vi "Free.vi"(8 "error in (no error)":errorcluster, 11 "Object (subject) in":refnum<class "Object (subject).lvclass">) -> (0 "error out":errorcluster, 3 "Object (subject) out":refnum<class "Object (subject).lvclass">)   [LabVIEW 2014, in "Object (subject).lvclass"]
uses:
  Object (subject).lvclass
  Object (subject).lvclass/Object (subject).ctl
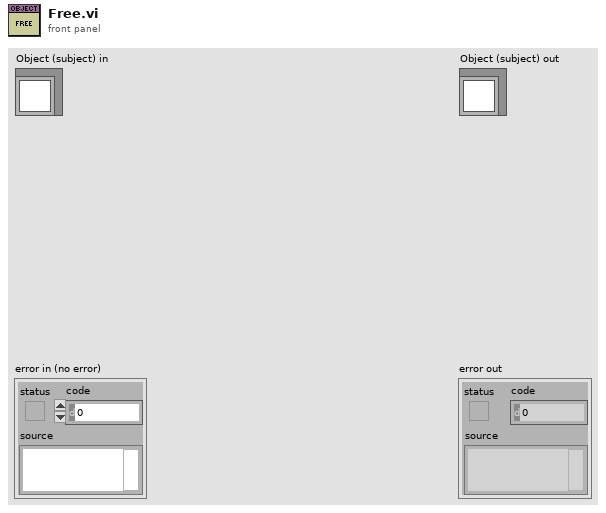
[diagram p1: front panel]
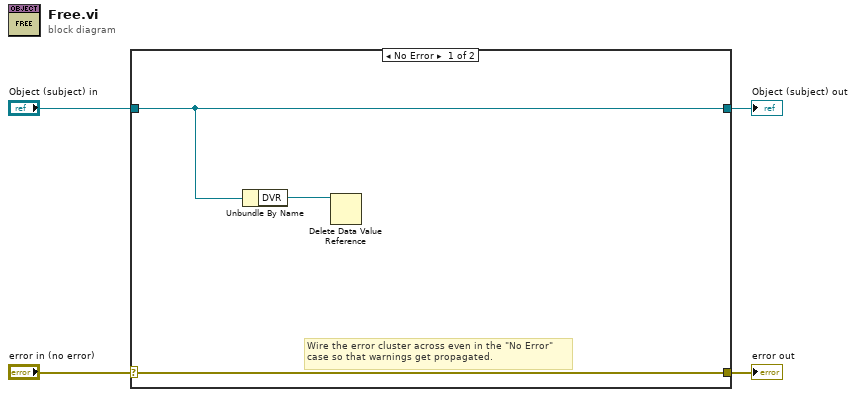
[diagram p0: block diagram]
diagram:
  n1 = case shown="No Error" "error in (no error)" {
    selector: "error in (no error)" -> [w7 w9]
    tunnel: [w7 w9] -> w3
    tunnel: [w6 w8] -> w1
    tunnel: "Object (subject) in" -> [w6 w8]
    frame No Error {
      # "Wire the error cluster across even in the \"No Error\"\ncase so that warnings get propagated."
      n2 = Unbundle By Name(w6) -> ("DVR"=w5:refnum<data-value>)
      n3 = Delete Data Value Reference(data value reference=w5) -> ()  [unwired: 1 in, 2 out]
    }
    frame Error {
    }
  }
  "error out" <- w3
  "Object (subject) out" <- w1
